vi "Script VeriStand Model for All Targets.vi"   [LabVIEW 2014]
uses:
  CD model script.lvlib
types:
  T1 = enum32{"Invalid", "Standard", "Closed", "Hidden", "Minimized", "Maximized"}
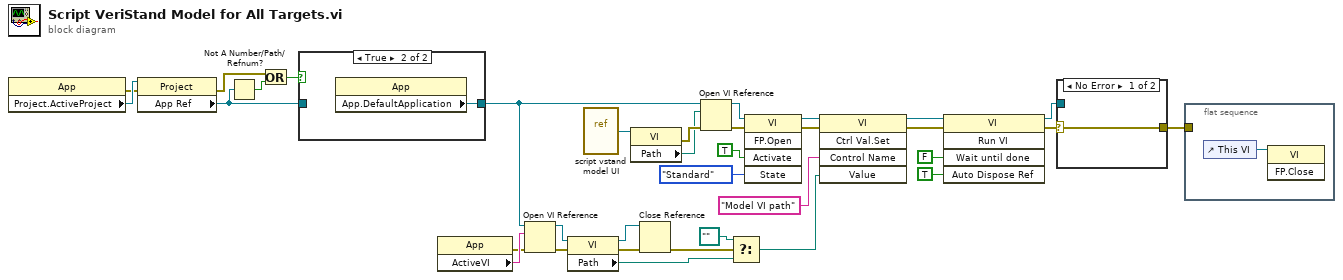
[diagram p0: block diagram]
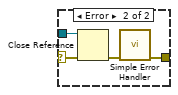
[diagram p3: hidden frame]
diagram:
  n1 = property class="App"() -> (error out=w33:errorcluster, "Project.ActiveProject"=w34:refnum<vi>)  [unwired: 2 in, 1 out]
  n2 = property class="Project"(reference=w34, error in=w33) -> (error out=w18:errorcluster, "App Ref"=w16:refnum<vi>)  [unwired: 1 out]
  n3 = Not A Number/Path/Refnum?(number/path/refnum=w16) -> (NaN/Path/Refnum?=w19:bool)
  n4 = Or(x=w18, y=w19) -> (x .or. y?=w17:bool)
  n5 = case shown="True" w17 {
    tunnel: [w35 w36] -> w11
    tunnel: w16 -> [w35 _]
    frame False {
    }
    frame True {
      n6 = property class="App"() -> ("App.DefaultApplication"=w36:refnum<vi>)  [unwired: 2 in, 2 out]
    }
  }
  n7 = property class="App"() -> (error out=w1:errorcluster, "ActiveVI"=w10:string)  [unwired: 2 in, 1 out]
  n8 = Open VI Reference(application reference (local)=w11, vi path=w10, error in (no error)=w1) -> (vi reference=w8:refnum<vi>, error out=w9:errorcluster)  [unwired: 3 in]
  n9 = property class="VI"(reference=w8, error in=w9) -> (reference out=w6:refnum<vi>, error out=w7:errorcluster, "Path"=w5:path)
  n10 = vi-ref "script vstand model UI.vi"() -> (w31:refnum<vi>)
  n11 = property class="VI"(reference=w31) -> (error out=w32:errorcluster, "Path"=w30:path)  [unwired: 1 in, 1 out]
  n12 = Close Reference(reference=w6, error in (no error)=w7) -> (error out=w2:errorcluster)
  n13 = Open VI Reference(application reference (local)=w11, vi path=w30, error in (no error)=w32) -> (vi reference=w29:refnum<vi>, error out=w28:errorcluster)  [unwired: 3 in]
  n14 = Select(t=path "", s=w2, f=w5) -> (s? t:f=w3:path)
  n15 = invoke class="VI" method="FP.Open"(reference=w29, error in=w28, "Activate"=TRUE ("Activate?"), "State"=T1."Standard") -> (reference out=w14:refnum<vi>, error out=w27:errorcluster)  [unwired: 1 in, 3 out]
  n16 = invoke class="VI" method="Ctrl Val.Set"(reference=w14, error in=w27, "Control Name"="Model VI path", "Value"=w3) -> (reference out=w13:refnum<vi>, error out=w15:errorcluster)  [unwired: 1 in, 3 out]
  n17 = invoke class="VI" method="Run VI"(reference=w13, error in=w15, "Wait until done"=FALSE ("Wait Until Done"), "Auto Dispose Ref"=TRUE ("Auto Dispose Reference")) -> (reference out=w25:refnum<vi>, error out=w26:errorcluster)  [unwired: 1 in, 3 out]
  n18 = case shown="No Error" w26 {
    selector: w26 -> [w37 w41]
    tunnel: w25 -> [_ w40]
    tunnel: [w37 w38] -> w20
    frame No Error {
    }
    frame Error {
      n19 = Close Reference(reference=w40, error in (no error)=w41) -> (error out=w39:errorcluster)
      n20 = call <vilib>:"Simple Error Handler.vi"("error in (no error)"=w39) -> ("error out"=w38:errorcluster)  [unwired: 4 in, 4 out]
    }
  }
  n21 = flat-sequence {
    tunnel: w20 -> [_]
    frame #0 {
      n22 = control-ref of="This VI"() -> (w42:refnum<vi>)
      n23 = invoke class="VI" method="FP.Close"(reference=w42) -> ()  [unwired: 2 in, 3 out]
    }
  }
